vi "Implement IIR Cascade Filter (DBL).vi"(7 "Reset":bool, 8 "error in (no error)":errorcluster, 10 "IIR Filter Cluster":T1 {"Forward Coefficients" format="%0.4f"; "Reverse Coefficients" format="%0.4f"}, 11 "Waveform":waveform(dbl)) -> (0 "error out":errorcluster, 3 "Filtered Waveform":waveform(dbl))   [LabVIEW 2020, in "NI_MAPro.lvlib"]
uses:
  NI_MAPro.lvlib
  NI_MABase.lvlib
  NI_AALBase.lvlib
panel:
  in  "shift register type":dbl[](array[numeric]) format="%0.2f"
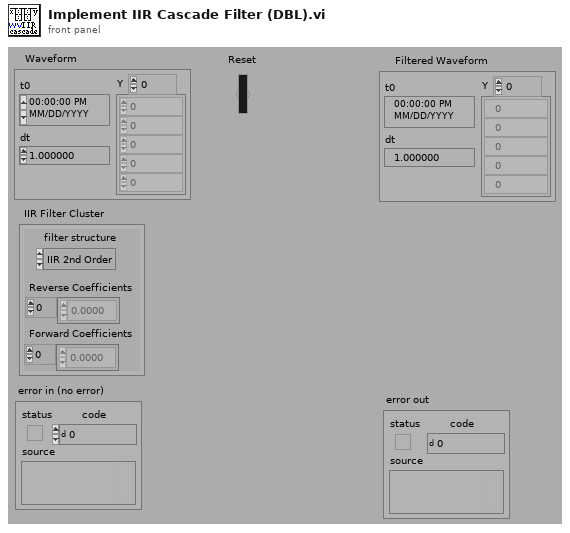
[diagram p1: front panel]
types:
  T1 = cluster{"filter structure":enum32{"IIR 2nd Order", "IIR 4th Order"}, "Reverse Coefficients":dbl[], "Forward Coefficients":dbl[]}
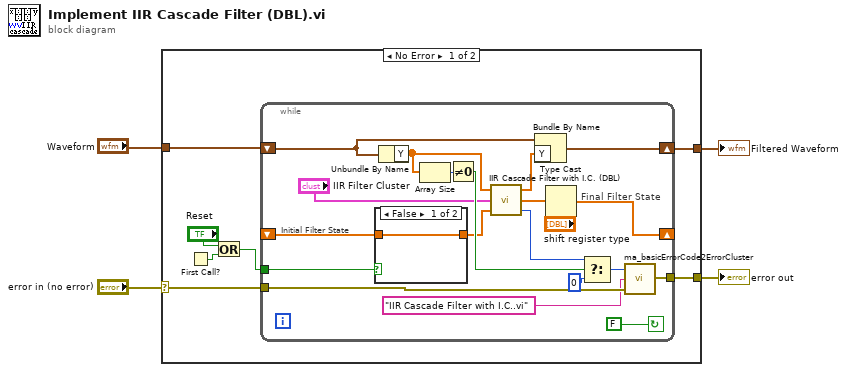
[diagram p0: block diagram]
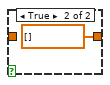
[diagram p2: hidden frame]
diagram:
  n1 = case shown="No Error" "error in (no error)" {
    selector: "error in (no error)" -> [w10 w35]
    tunnel: [w11 w35] -> w3
    tunnel: [w9 w34] -> w2
    tunnel: "Waveform" -> [w8 w34]
    frame No Error {
      n2 = First Call?() -> (First Call?: T/F=w5:bool)
      n3 = Or(x="Reset", y=w5) -> (x .or. y?=w6:bool)
      n4 = while {
        tunnel: w10 -> [w18]
        tunnel: w6 -> [w20]
        tunnel: [w19] -> w11
        shift-left: w8 -> [w26]
        shift-right: [w27] -> w9
        shift-left: _ -> [w22]
        shift-right: [w30] -> _
        stop <- FALSE continue-if-true
        # "Final Filter State"
        # "Initial Filter State"
        n5 = case shown="False" w20 {
          tunnel: w22 -> [w32 _]
          tunnel: [w32 dbl[] [] ("shift register type")] -> w21
          frame False {
          }
          frame True {
          }
        }
        n6 = Unbundle By Name(w26) -> ("Y"=w13:dbl[])
        n7 = Array Size(array=w13) -> (size(s)=w12:i32)
        n8 = Not Equal To 0?(x=w12) -> (x != 0?=w31:bool)
        n9 = call "IIR Cascade Filter with I.C. (DBL).vi"("Initial Filter State"=w21, "IIR Filter Cluster"="IIR Filter Cluster", "X"=w13) -> ("error"=w14:i32, "Final Filter State"=w23:dbl[], "Filtered X"=w25:dbl[])
        n10 = Bundle By Name(cluster=w26, "Y"=w25) -> (w27:waveform(dbl))
        n11 = Type Cast(type="shift register type", x=w23) -> (*(type *) &x=w30:dbl[])
        n12 = Select(t=w14, s=w31, f=0) -> (s? t:f=w15:i32)
        n13 = call "ma_basicErrorCode2ErrorCluster.vi"("error in (no error)"=w18, "subVI name"="IIR Cascade Filter with I.C..vi", "Error Code"=w15) -> ("error out"=w19:errorcluster)
      }
    }
    frame Error {
    }
  }
  "error out" <- w3
  "Filtered Waveform" <- w2
